vi "Truncate Value String End.vi"(10 "Value String In":string caption="数值字符串输入") -> (2 "Value String Out":string caption="数值字符串输出")   [LabVIEW 2023, in "Longer Pump dLSP501 Series.lvlib"]
uses:
  <instrlib>/Longer Pump dLSP501 Modbus RTU Series/Longer Pump dLSP501 Series.lvlib
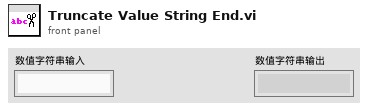
[diagram p1: front panel]
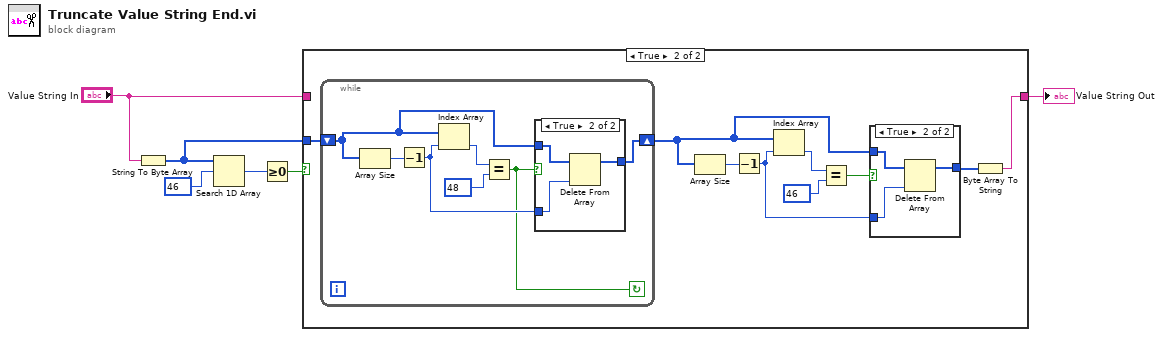
[diagram p0: block diagram]
diagram:
  n1 = String To Byte Array(string="Value String In") -> (unsigned byte array=w1:u8[])
  n2 = Search 1D Array(1D array=w1, element=46) -> (index of element=w5:i32)  [unwired: 1 in]
  n3 = Greater Or Equal To 0?(x=w5) -> (x >= 0?=w4:bool)
  n4 = case shown="True" w4 {
    tunnel: "Value String In" -> [w7 _]
    tunnel: [w7 w15] -> w2
    tunnel: w1 -> [_ w16]
    frame False {
    }
    frame True {
      n5 = while {
        shift-right: [w22] -> w9
        shift-left: w16 -> [w24]
        stop <- w21 continue-if-true
        n6 = Array Size(array=w24) -> (size(s)=w27:i32)
        n7 = Decrement(x=w27) -> (x-1=w23:i32)
        n8 = Index Array(array=w24, index=w23) -> (element=w26:u8)
        n9 = Equal?(x=w26, y=48) -> (x = y?=w21:bool)
        n10 = case shown="True" w21 {
          tunnel: w24 -> [w28 w31]
          tunnel: w23 -> [_ w30]
          tunnel: [w28 w29] -> w22
          frame False {
          }
          frame True {
            n11 = Delete From Array(array=w31, index=w30) -> (array with subset deleted=w29:u8[])  [unwired: 1 in, 1 out]
          }
        }
      }
      n12 = Array Size(array=w9) -> (size(s)=w14:i32)
      n13 = Decrement(x=w14) -> (x-1=w11:i32)
      n14 = Index Array(array=w9, index=w11) -> (element=w13:u8)
      n15 = Equal?(x=w13, y=46) -> (x = y?=w10:bool)
      n16 = case shown="True" w10 {
        tunnel: w9 -> [w17 w20]
        tunnel: w11 -> [_ w19]
        tunnel: [w17 w18] -> w8
        frame False {
        }
        frame True {
          n17 = Delete From Array(array=w20, index=w19) -> (array with subset deleted=w18:u8[])  [unwired: 1 in, 1 out]
        }
      }
      n18 = Byte Array To String(unsigned byte array=w8) -> (string=w15:string)
    }
  }
  "Value String Out" <- w2
